vi "温度湿度最大值最小值.vi"(6 "湿度移位寄存器输入":dbl[](array[numeric]), 9 "输出簇":T1, 10 "温度移位寄存器输入":dbl[](array[numeric]), 11 "循环计数":dbl) -> (1 "湿度最大值":dbl, 2 "温度最大值":dbl, 3 "温度最小值":dbl, 4 "湿度最小值":dbl, 5 "湿度移位寄存器输出":dbl[](array[numeric]), 7 "温度移位寄存器输出":dbl[](array[numeric]))   [LabVIEW 2012]
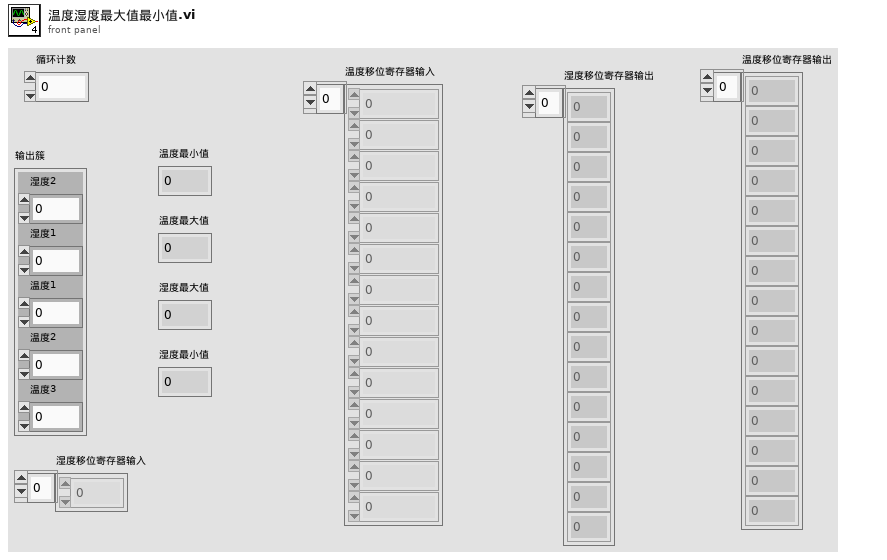
[diagram p1: front panel]
types:
  T1 = cluster{"湿度2":dbl, "湿度1":dbl, "温度1":dbl, "温度2":dbl, "温度3":dbl}
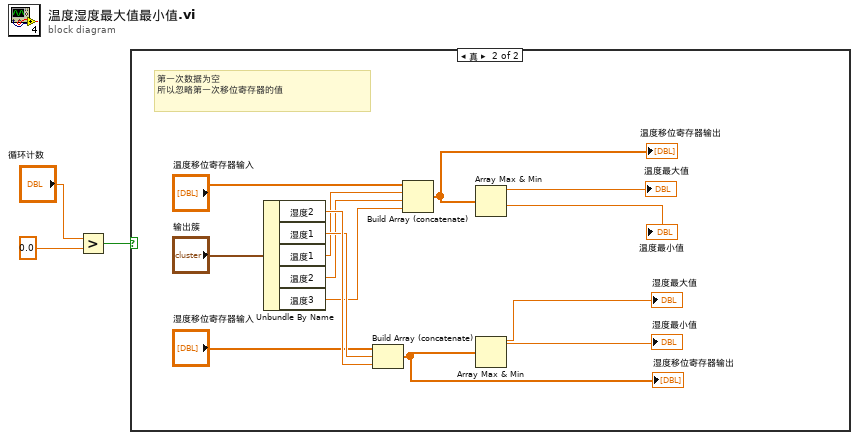
[diagram p0: block diagram]
diagram:
  n1 = Greater?(x="循环计数", y=0.0) -> (0:w2:bool)
  n2 = case shown="真" w2 {
    frame False {
    }
    frame True {
      # "第一次数据为空\n所以忽略第一次移位寄存器的值"
      n3 = Unbundle By Name("输出簇") -> ("湿度2"=w14:dbl, "湿度1"=w13:dbl, "温度1"=w7:dbl, "温度2"=w8:dbl, "温度3"=w9:dbl)
      n4 = Build Array (concatenate)("湿度移位寄存器输入", w13, w14) -> (w17:dbl[])
      "湿度移位寄存器输出" <- w17
      n5 = Build Array (concatenate)("温度移位寄存器输入", w7, w8, w9) -> (w4:dbl[])
      "温度移位寄存器输出" <- w4
      n6 = Array Max & Min(array=w4) -> (max value=→"温度最大值":dbl, min value=→"温度最小值":dbl)  [unwired: 2 out]
      n7 = Array Max & Min(array=w17) -> (max value=→"湿度最大值":dbl, min value=→"湿度最小值":dbl)  [unwired: 2 out]
    }
  }
